vi "blob open.vi"(0 "para0":dbl, 1 "iRow":u64, 2 "ppBlob":dbl, 5 "zDb":string, 7 "zTable":string, 9 "zColumn":string, 11 "error in (no error)":errorcluster, 12 "flags":i32) -> (4 "para0 out":dbl, 6 "ppBlob out":dbl, 8 "function return":i32, 15 "error out":errorcluster)   [LabVIEW 2020, in "sqlite3.lvlib"]
uses:
  sqlite3.lvlib
  errstr.vi
  bin/sqlite3_64.dll
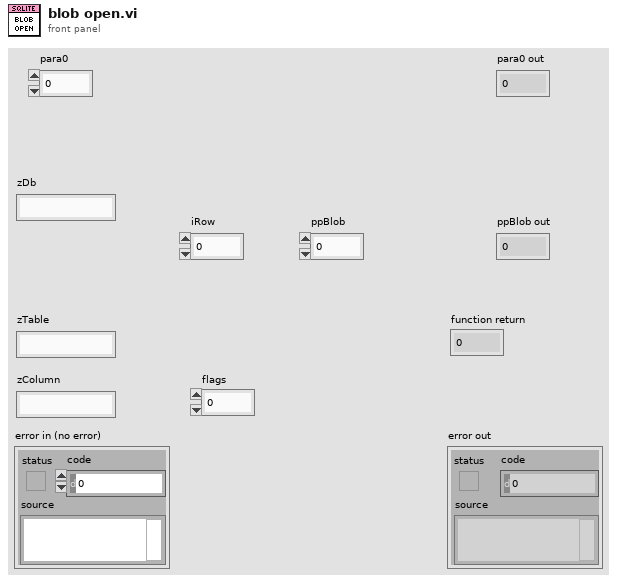
[diagram p1: front panel]
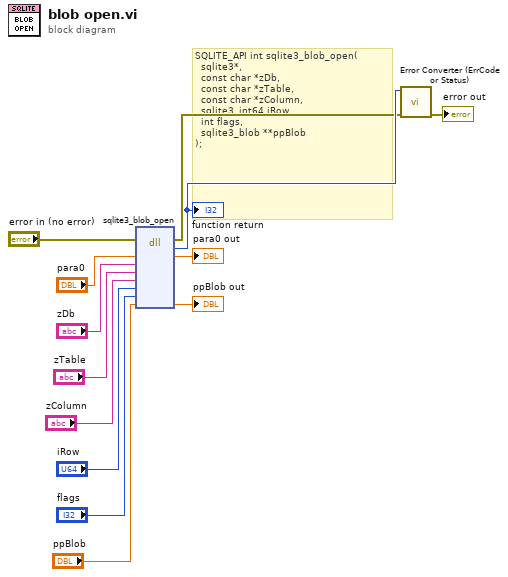
[diagram p0: block diagram]
diagram:
  # "SQLITE_API int sqlite3_blob_open(\n  sqlite3*,\n  const char *zDb,\n  const char *zTable,\n  const char *zColumn,\n  sqlite3_int64 iRow,\n  int flags,\n  sqlite3_blob **ppBlob\n);"
  n1 = dll-call lib="C:/Users/Fred.Guo/Desktop/Database-configuration/externals/sqlite3/Source/bin/sqlite3_*.*" fn="sqlite3_blob_open"(error in="error in (no error)", "para0"="para0", "zDb"="zDb", "zTable"="zTable", "zColumn"="zColumn", "iRow"="iRow", "flags"="flags", "ppBlob"="ppBlob") -> (error out=w2:errorcluster, w13:i32, "para0"=→"para0 out":dbl, "ppBlob"=→"ppBlob out":dbl)  [unwired: 7 in, 1 out]
  "function return" <- w13
  n2 = call "Error Converter (ErrCode or Status).vi"("error in (no error)"=w2, "error code"=w13) -> ("error out"=→"error out":errorcluster)  [unwired: 9 in]
